vi "Write Objects.vi"(8 "error in (no error)":errorcluster, 10 "objects":T1[](array[typedef]) {"Object ID" format="%x"}, 11 "standard data model in":refnum<class "ELAN Data Model.lvclass">) -> (0 "error out":errorcluster, 3 "standard data model out":refnum<class "ELAN Data Model.lvclass">)   [LabVIEW 2021, in "ELAN Data Model.lvclass"]
doc: "Writes objects to the device model."
uses:
  ELAN Data Model.lvclass
  Modbus_v121c/Data Model/Identification Parameters.ctl
  ELAN Data Model.lvclass/ELAN Data Model.ctl
  Modbus_v121c/Data Model/Device Data Model.lvclass
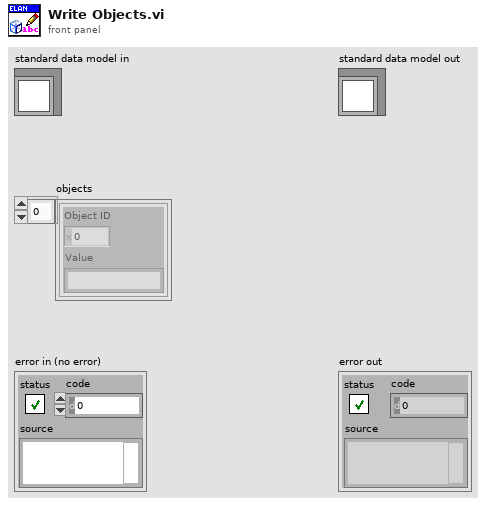
[diagram p1: front panel]
types:
  T1 = typedef "Device Data Model.lvclass/Identification Parameters.ctl" = cluster{"Object ID":u8, "Value":string}
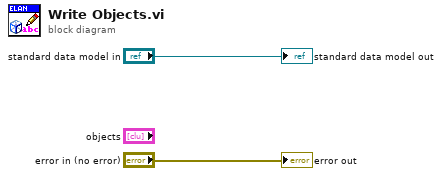
[diagram p0: block diagram]
diagram:
  "error out" <- "error in (no error)"
  "standard data model out" <- "standard data model in"
